vi "Create Evaluations.vi"(8 "error in (no error)":errorcluster, 11 "IEvaluation in":refnum<class "IMD_ACP.lvclass">) -> (0 "error out":errorcluster, 2 "Evaluations Out":T1[](array[typedef]) {"Low Limit" format="%#_13g"; "SI Scaling" items=["femto"=-15, "pico"=-12, "nano"=-9, "micro"=-6, "milli"=-3, "percent"=-2, ""=0, "kilo"=3, "mega"=6, "giga"=9, "tera"=12]}, 3 "IEvaluation out":refnum<class "IMD_ACP.lvclass">)   [LabVIEW 2018, in "SeqAuto Evaluations.lvlib" / "IMD_ACP.lvclass"]
uses:
  IMD_ACP.lvclass
  C:/Sequence Automation/Plugins/SeqAuto IEvaluation.lvlibp/SeqAuto IEvaluation.lvclass
  Plugins/TestStand API Tools (TSAT).lvlibp/Evaluation Actions/Includes/Controls/TSAT Evaluation.ctl
  Plugins/TestStand API Tools (TSAT).lvlibp/Evaluation Actions/Includes/Controls/TSAT Eval SI Unit Scaling.ctl
  Plugins/TestStand API Tools (TSAT).lvlibp/Evaluation Actions/Includes/Controls/TSAT Evaluation Type.ctl
  IMD_ACP.lvclass/IMD_ACP.ctl
  Read SA Pin.vi
  Read Signal Suffix.vi
  Plugins/SeqAuto IEvaluation.lvlibp/Read Measurement Name.vi
  Plugins/TestStand API Tools (TSAT).lvlibp/Evaluation Actions/TSAT Evaluation Actions.lvlib
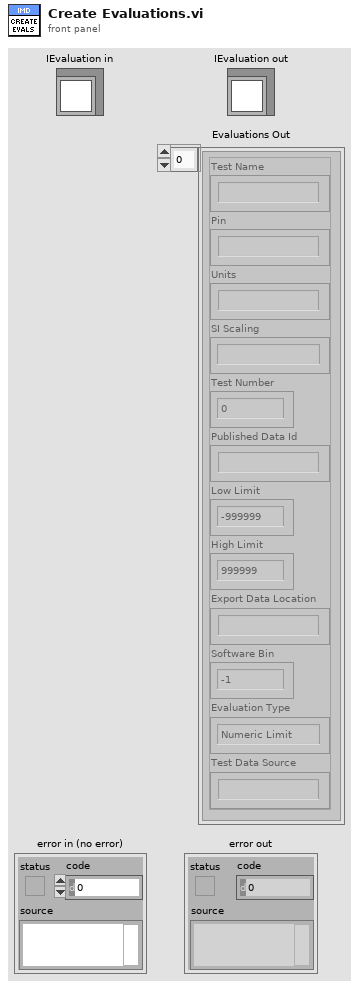
[diagram p1: front panel]
types:
  T1 = typedef "TestStand API Tools (TSAT).lvlibp/TSAT Evaluation Actions.lvlib/TSAT Evaluation.ctl" = cluster{"Test Name":string, "Pin":string, "Units":string, "SI Scaling":T2, "Test Number":i32, "Published Data Id":string, "Low Limit":dbl, "High Limit":dbl, "Export Data Location":string, "Software Bin":i64, "Evaluation Type":T3, "Test Data Source":string}
  T2 = typedef "TestStand API Tools (TSAT).lvlibp/TSAT Evaluation Actions.lvlib/TSAT Eval SI Unit Scaling.ctl" = i16
  T3 = typedef "TestStand API Tools (TSAT).lvlibp/TSAT Evaluation Actions.lvlib/TSAT Evaluation Type.ctl" = enum16{"Numeric Limit", "Pass/Fail", "None"}
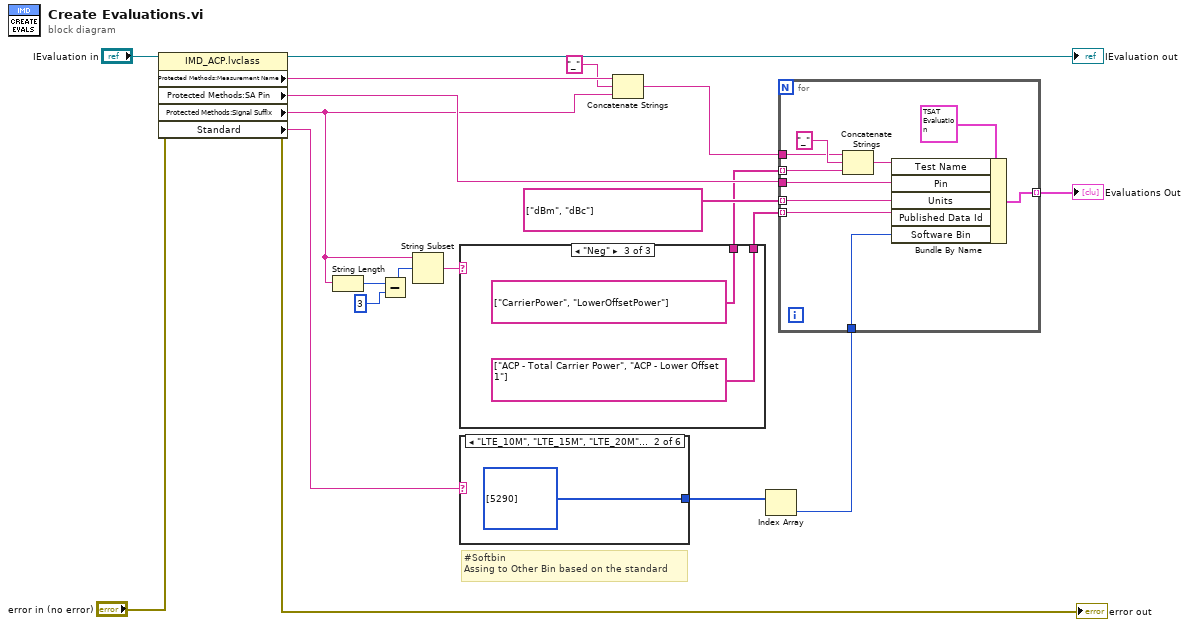
[diagram p0: block diagram]
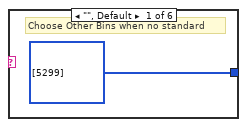
[diagram p2: hidden frame]
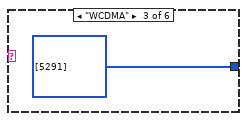
[diagram p3: hidden frame]
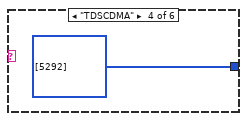
[diagram p4: hidden frame]
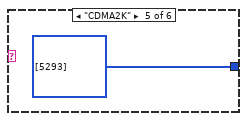
[diagram p5: hidden frame]
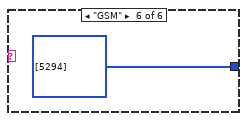
[diagram p6: hidden frame]
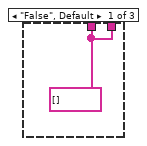
[diagram p7: hidden frame]
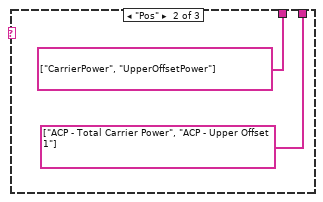
[diagram p8: hidden frame]
diagram:
  # "#Softbin\nAssing to Other Bin based on the standard"
  n1 = property class="IMD_ACP.lvclass"(reference="IEvaluation in", error in="error in (no error)") -> (reference out=→"IEvaluation out":refnum<class "IMD_ACP.lvclass">, error out=→"error out":errorcluster, "Protected Methods:Measurement Name"=w18:string, "Protected Methods:SA Pin"=w17:string, "Protected Methods:Signal Suffix"=w3:string, "Standard"=w5:string)
  n2 = String Length(string=w3) -> (length=w13:i32)
  n3 = Subtract(x=w13, y=3) -> (x-y=w11:i32)
  n4 = String Subset(string=w3, offset (0)=w11) -> (substring=w10:string)  [unwired: 1 in]
  n5 = case shown="\"Neg\"" w10 {
    tunnel: [w21 string[] ["ACP - Total Carrier Power", "ACP - Upper Offset 1"] string[] ["ACP - Total Carrier Power", "ACP - Lower Offset 1"]] -> w15
    tunnel: [w21 string[] ["CarrierPower", "UpperOffsetPower"] string[] ["CarrierPower", "LowerOffsetPower"]] -> w1
    frame "False", Default {
      w21 = string[] []
    }
    frame "Pos" {
    }
    frame "Neg" {
    }
  }
  n6 = case shown="\"LTE_10M\", \"LTE_15M\", \"LTE_20M\", \"LTE_30M\", \"LTE_40M\"" w5 {
    tunnel: [i64[] [5299] i64[] [5290] i64[] [5291] i64[] [5292] i64[] [5293] i64[] [5294]] -> w7
    frame "", Default {
      # "Choose Other Bins when no standard"
    }
    frame "LTE_10M", "LTE_15M", "LTE_20M", "LTE_30M", "LTE_40M" {
    }
    frame "WCDMA" {
    }
    frame "TDSCDMA" {
    }
    frame "CDMA2K" {
    }
    frame "GSM" {
    }
  }
  n7 = Concatenate Strings(w18, "_" ("string"), w3) -> (w4:string)
  n8 = Index Array(array=w7) -> (element=w6:i64)  [unwired: 1 in]
  n9 = for {
    tunnel: [w40] -> w14 mode=indexing
    tunnel: w4 -> [w32]
    tunnel: w17 -> [w39]
    tunnel: string[] ["dBm", "dBc"] -> [w38] mode=indexing
    tunnel: w15 -> [w37] mode=indexing
    tunnel: w6 -> [w36]
    tunnel: w1 -> [w34] mode=indexing
    n10 = Concatenate Strings(w32, "_" ("string"), w34) -> (w33:string)
    n11 = Bundle By Name(cluster=T1 {"Test Name"="", "Pin"="", "Units"="", "SI Scaling"=0, "Test Number"=0, "Published Data Id"="", "Low Limit"=-999999.0, "High Limit"=999999.0, "Export Data Location"="", "Software Bin"=-1, "Evaluation Type"=enum."Numeric Limit", "Test Data Source"=""} ("Evaluation"), "Test Name"=w33, "Pin"=w39, "Units"=w38, "Published Data Id"=w37, "Software Bin"=w36) -> (w40:T1)
  }
  "Evaluations Out" <- w14
